vi "configure g1(SCAPE) waveform.vi"(6 "error in (no error)":errorcluster, 8 "VISA resource name":refnum<visa-resource-name>="USB0::0x1AB1::0x0641::DG4E223801593::INSTR", 9 "enable":bool=TRUE, 10 "Output Channel (1: Channel 1)":i32(ring)=1 items=["Channel 1"=1, "Channel 2"=2], 11 "output cluster":T1={"waveform"=array[1024 elements], "Amplitude [Vpp]"=1.7319902098770545, "Frequency [Hz]"=50.0}) -> (0 "error out":errorcluster)   [LabVIEW 2024]
doc: "This example shows how to create then configure an arbitrary waveform."
uses:
  RIGOL DG4000 Series.lvlib
panel:
  # "(c) 2012 National Instruments.  ALL RIGHTS RESERVED."
  # "To edit the Arbitrary Waveform, use the Simulate Arbitrary Signal on the block diagram."
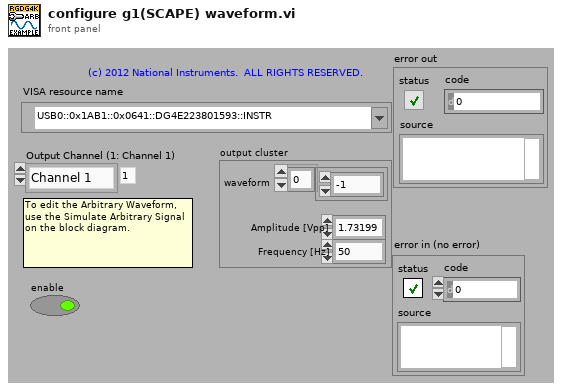
[diagram p1: front panel]
types:
  T1 = cluster{"waveform":dbl[], "Amplitude [Vpp]":dbl, "Frequency [Hz]":dbl}
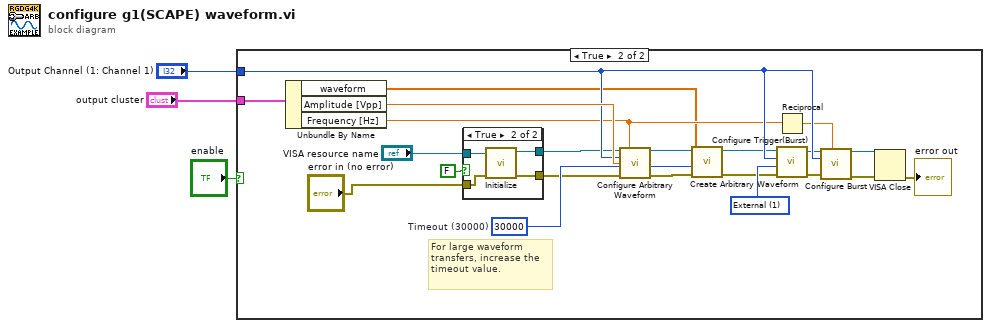
[diagram p0: block diagram]
diagram:
  n1 = case shown="True" "enable" {
    tunnel: "output cluster" -> [_ w22]
    tunnel: "Output Channel (1: Channel 1)" -> [_ w20]
    frame False {
    }
    frame True {
      w17 = 1 items=["Internal", "External", "Manual"] ("Trigger Source (0: Internal)")
      w24 = u32 30000  # Timeout (30000)
      # "For large waveform transfers, increase the timeout value."
      n2 = Unbundle By Name(w22) -> ("waveform"=w12:dbl[], "Amplitude [Vpp]"=w21:dbl, "Frequency [Hz]"=w14:dbl)
      n3 = case shown="True" FALSE {
        tunnel: "VISA resource name" -> [w27 w31]
        tunnel: [w26 w30] -> w7
        tunnel: [w27 w29] -> w9
        tunnel: "error in (no error)" -> [w26 w28]
        frame False {
        }
        frame True {
          n4 = call "Initialize.vi"("error in (no error)"=w28, "VISA resource name"=w31) -> ("error out"=w30:errorcluster, "VISA resource name out"=w29:refnum<visa-resource-name>)  [unwired: 2 in, 6 out]
        }
      }
      n5 = call "Configure Arbitrary Waveform.vi"("VISA resource name"=w9, "Frequency (1000 Hz)"=w14, "Output Channel (1: Channel 1)"=w20, "Amplitude (5 Vpp)"=w21, "error in (no error)"=w7) -> ("VISA resource name out"=w8:refnum<visa-resource-name>, "error out"=w6:errorcluster)  [unwired: 9 in]
      n6 = call "Create Arbitrary Waveform.vi"("error in (no error)"=w6, "Timeout (10000 ms)"=w24, "Arbitrary Waveform Data (0)"=w12, "VISA resource name"=w8) -> ("error out"=w4:errorcluster, "VISA resource name out"=w5:refnum<visa-resource-name>)  [unwired: 2 in, 4 out]
      n7 = Reciprocal(x=w14) -> (1/x=w13:dbl)
      n8 = call "Configure Trigger(Burst).vi"("error in (no error)"=w4, "Trigger Source (0: Internal)"=w17, "Trigger Channel (1: Channel 1)"=w20, "VISA resource name"=w5) -> ("error out"=w18:errorcluster, "VISA resource name out"=w19:refnum<visa-resource-name>)  [unwired: 6 in]
      n9 = call "Configure Burst.vi"("VISA resource name"=w19, "Burst Channel (1: Channel 1)"=w20, "error in (no error)"=w18, "Burst Period (0.01 s)"=w13) -> ("VISA resource name out"=w16:refnum<visa-resource-name>, "error out"=w15:errorcluster)  [unwired: 10 in]
      n10 = VISA Close(VISA resource name=w16, error in (no error)=w15) -> (error out=→"error out":errorcluster)
    }
  }
